vi "WCA_YTO_c_tune.vi"(0 "ObjHandle in":u32, 1 "SET YTO COARSE TUNE":sgl min=0 max=42 step=0.0001 format="%.4f", 2 "YTO Low freq. [GHz]":sgl=12.17 format="%.3f", 3 "YTO High freq. [GHz]":sgl=14.833 format="%.3f", 5 "error in (no error)":errorcluster, 8 "LO locked?":bool, 10 "Slave Node in":cluster{"Address":i16, "Serial Number":i8[]}={"Address"=19, "Serial Number"=[16, 71, 55, 76, 1, 8, 0, -15]} {"Serial Number" format="%.0x"; "Address" format="%.0x"}, 12 "Cartridge band":u32 max=10 step=1) -> (14 "ObjHandle out":u32, 19 "error out":errorcluster)   [LabVIEW 2017]
panel:
  out "YTOSet":u16
  # "Node Address"
  # "Serial Number"
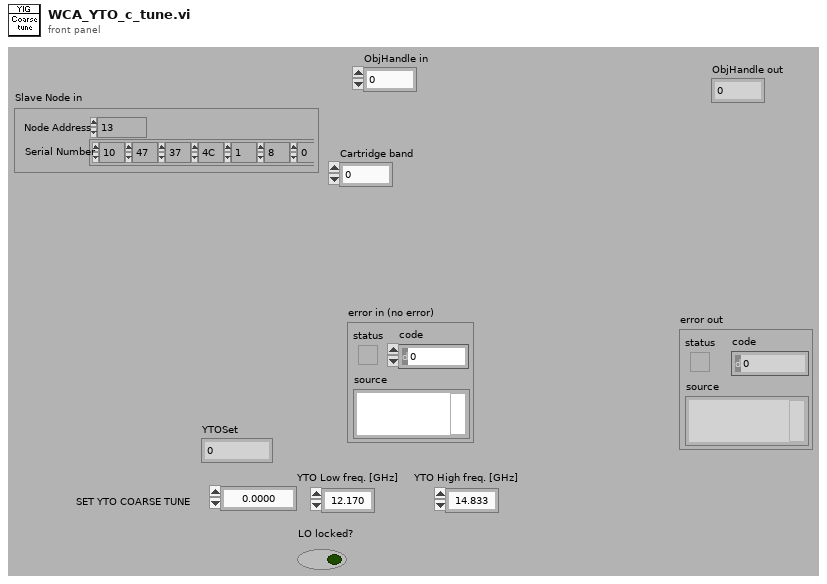
[diagram p1: front panel]
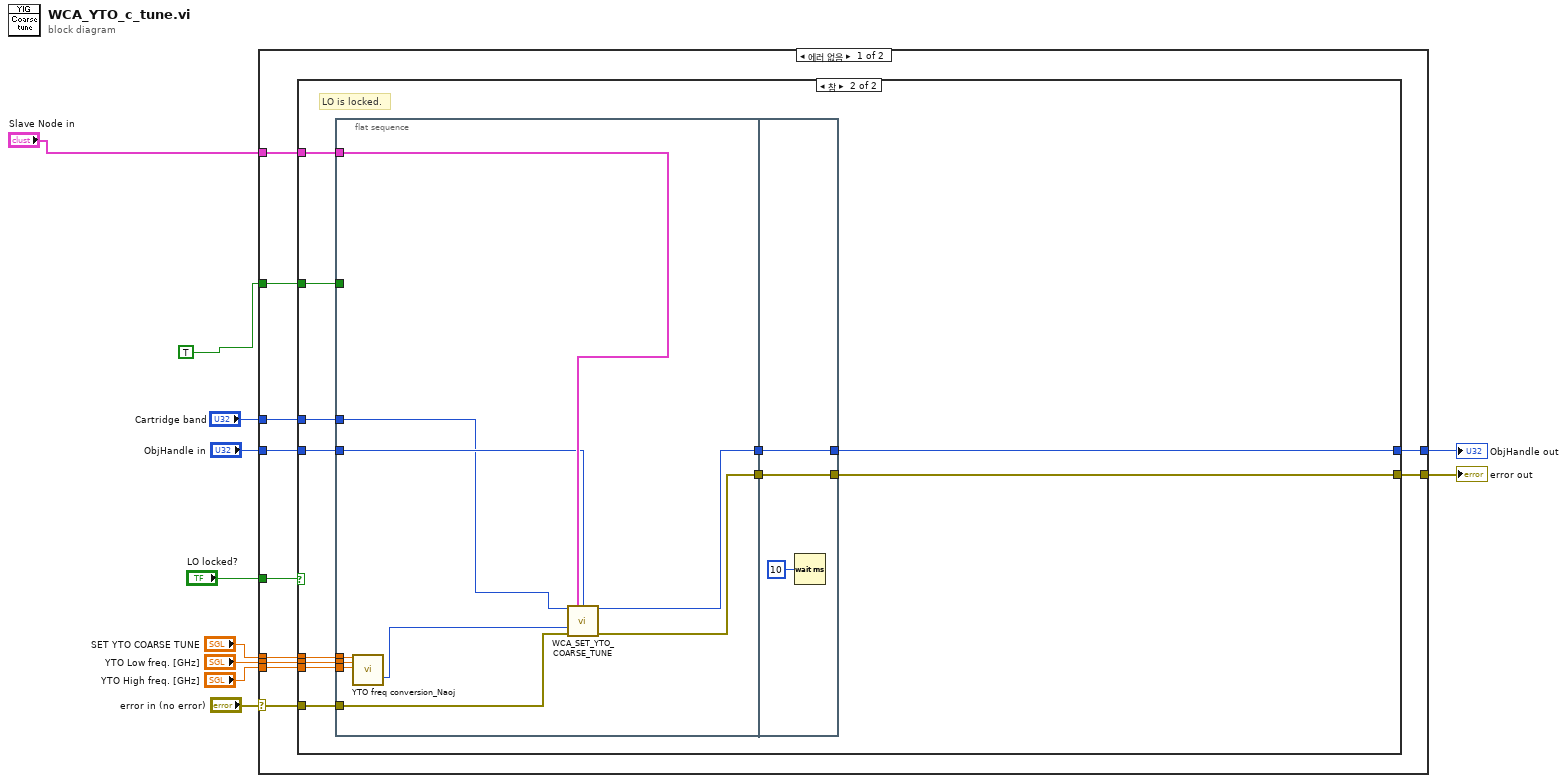
[diagram p0: block diagram]
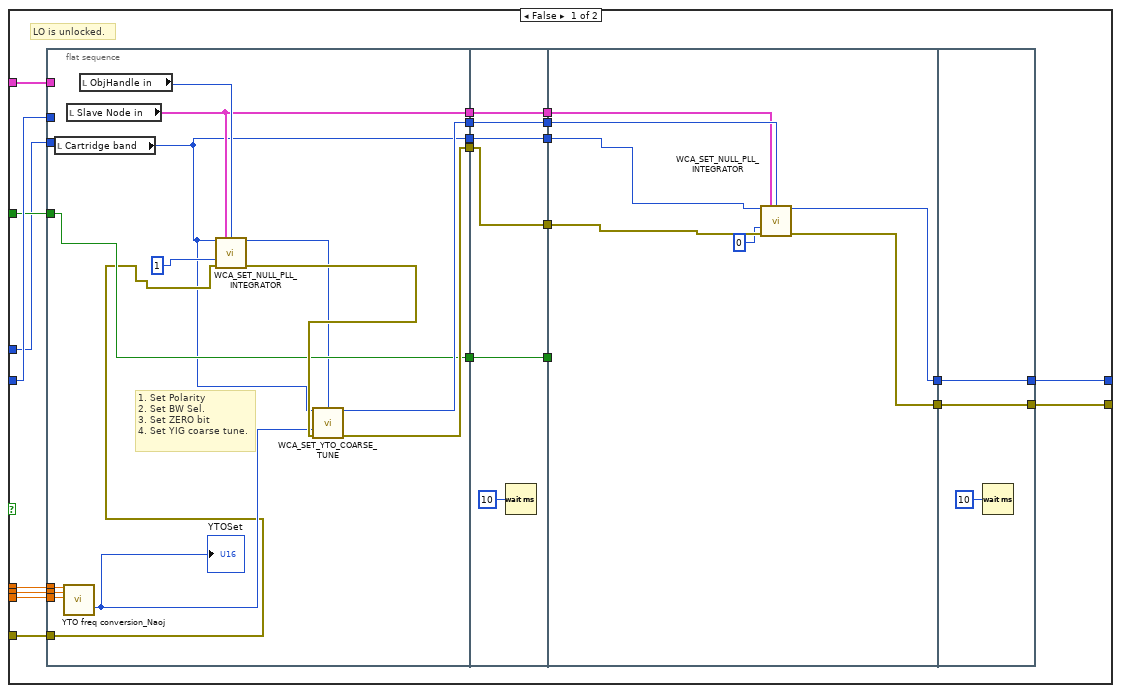
[diagram p2: hidden frame]
diagram:
  n1 = case shown="에러 없음" "error in (no error)" {
    selector: "error in (no error)" -> [w22 w101]
    tunnel: "ObjHandle in" -> [w21 w100]
    tunnel: "Slave Node in" -> [w20 _]
    tunnel: "SET YTO COARSE TUNE" -> [w19 _]
    tunnel: "YTO Low freq. [GHz]" -> [w18 _]
    tunnel: "YTO High freq. [GHz]" -> [w17 _]
    tunnel: TRUE -> [w16 _]
    tunnel: [w15 w101] -> w6
    tunnel: [w14 w100] -> w5
    tunnel: "LO locked?" -> [w13 _]
    tunnel: "Cartridge band" -> [w12 _]
    frame No Error {
      n2 = case shown="참" w13 {
        tunnel: w22 -> [w42 w84]
        tunnel: w21 -> [w41 w83]
        tunnel: w20 -> [w40 w82]
        tunnel: w19 -> [w39 w81]
        tunnel: w18 -> [w38 w80]
        tunnel: w17 -> [w37 w79]
        tunnel: w16 -> [w36 w78]
        tunnel: [w35 w76] -> w15
        tunnel: [w34 w77] -> w14
        tunnel: w12 -> [w33 w75]
        frame False {
          # "LO is unlocked."
          n3 = flat-sequence {
            tunnel: w42 -> [w50]
            tunnel: w41 -> [_]
            tunnel: w40 -> [_]
            tunnel: w39 -> [w58]
            tunnel: w38 -> [w57]
            tunnel: w37 -> [w56]
            tunnel: w36 -> [w51]
            tunnel: w33 -> [_]
            tunnel: [w54] -> w32
            tunnel: [w53] -> w29
            tunnel: [w51] -> w28
            tunnel: [w46] -> w26
            tunnel: [w45] -> w24
            tunnel: w32 -> [w63]
            tunnel: [w63] -> w31
            tunnel: [w62] -> w30
            tunnel: w29 -> [w62]
            tunnel: w28 -> [w61]
            tunnel: [w61] -> w27
            tunnel: w26 -> [w60]
            tunnel: [w60] -> w25
            tunnel: w24 -> [w59]
            tunnel: [w59] -> w23
            tunnel: [w69] -> w44
            tunnel: [w68] -> w43
            tunnel: w31 -> [w71]
            tunnel: w30 -> [w70]
            tunnel: w27 -> [_]
            tunnel: w25 -> [w66]
            tunnel: w23 -> [w65]
            tunnel: [w73] -> w35
            tunnel: w44 -> [w73]
            tunnel: [w72] -> w34
            tunnel: w43 -> [w72]
            frame #0 {
              # "1. Set Polarity\n2. Set BW Sel.\n3. Set ZERO bit\n4. Set YIG coarse tune."
              n4 = local read "Cartridge band"() -> (w45:u32)
              n5 = call "YTO freq conversion_Naoj.vi"("YTO desired frequency"=w58, "YTO freq Min"=w57, "YTO freq. Max"=w56) -> ("YTO Coarse tune"=w52:u16)  [unwired: 16 in]
              "YTOSet" <- w52
              n6 = local read "Slave Node in"() -> (w46:cluster{"Address":i16, "Serial Number":i8[]})
              n7 = local read "ObjHandle in"() -> (w47:u32)
              n8 = call "WCA_SET_NULL_PLL_INTEGRATOR.vi"("Cartridge Band"=w45, "Slave Node in"=w46, "ObjHandle in"=w47, "SET_NULL_PLL_INTEGRATOR"=1 ("SET NULL PLL INTEGRATOR"), "error in (no error)"=w50) -> ("ObjHandle out"=w48:u32, "error out"=w55:errorcluster)  [unwired: 9 in]
              n9 = call "WCA_SET_YTO_COARSE_TUNE.vi"("Cartridge Band"=w45, "ObjHandle in"=w48, "SET_YTO_COARSE_TUNE"=w52, "error in (no error)"=w55) -> ("ObjHandle out"=w54:u32, "error out"=w53:errorcluster)  [unwired: 10 in]
            }
            frame #1 {
              n10 = Wait (ms)(milliseconds to wait=u32 10) -> ()  [unwired: 1 out]
            }
            frame #2 {
              n11 = call "WCA_SET_NULL_PLL_INTEGRATOR.vi"("Cartridge Band"=w65, "Slave Node in"=w66, "ObjHandle in"=w71, "SET_NULL_PLL_INTEGRATOR"=0 ("SET NULL PLL INTEGRATOR"), "error in (no error)"=w70) -> ("ObjHandle out"=w68:u32, "error out"=w69:errorcluster)  [unwired: 9 in]
            }
            frame #3 {
              n12 = Wait (ms)(milliseconds to wait=u32 10) -> ()  [unwired: 1 out]
            }
          }
        }
        frame True {
          # "LO is locked."
          n13 = flat-sequence {
            tunnel: w84 -> [w88]
            tunnel: w83 -> [w90]
            tunnel: w82 -> [w91]
            tunnel: w81 -> [w96]
            tunnel: w80 -> [w95]
            tunnel: w79 -> [w94]
            tunnel: w78 -> [_]
            tunnel: [w92] -> w86
            tunnel: [w87] -> w85
            tunnel: w75 -> [w89]
            tunnel: w86 -> [w98]
            tunnel: w85 -> [w97]
            tunnel: [w98] -> w77
            tunnel: [w97] -> w76
            frame #0 {
              n14 = call "YTO freq conversion_Naoj.vi"("YTO desired frequency"=w96, "YTO freq Min"=w95, "YTO freq. Max"=w94) -> ("YTO Coarse tune"=w93:u16)  [unwired: 16 in]
              n15 = call "WCA_SET_YTO_COARSE_TUNE.vi"("Cartridge Band"=w89, "Slave Node in"=w91, "ObjHandle in"=w90, "SET_YTO_COARSE_TUNE"=w93, "error in (no error)"=w88) -> ("ObjHandle out"=w92:u32, "error out"=w87:errorcluster)  [unwired: 9 in]
            }
            frame #1 {
              n16 = Wait (ms)(milliseconds to wait=u32 10) -> ()  [unwired: 1 out]
            }
          }
        }
      }
    }
    frame Error {
    }
  }
  "error out" <- w6
  "ObjHandle out" <- w5
